vi "Read Protocol ID.vi"(8 "error in (no error)":errorcluster, 11 "MB_ADU_TCP in":refnum<class "MB_ADU_TCP.lvclass">) -> (0 "error out":errorcluster, 2 "Protocol ID":u16, 3 "MB_ADU_TCP out":refnum<class "MB_ADU_TCP.lvclass">)   [LabVIEW 2012, in "MB Master.lvlib" / "MB_ADU_TCP.lvclass"]
uses:
  MB_ADU_TCP.lvclass
  MB_ADU_TCP.lvclass/MB_ADU_TCP.ctl
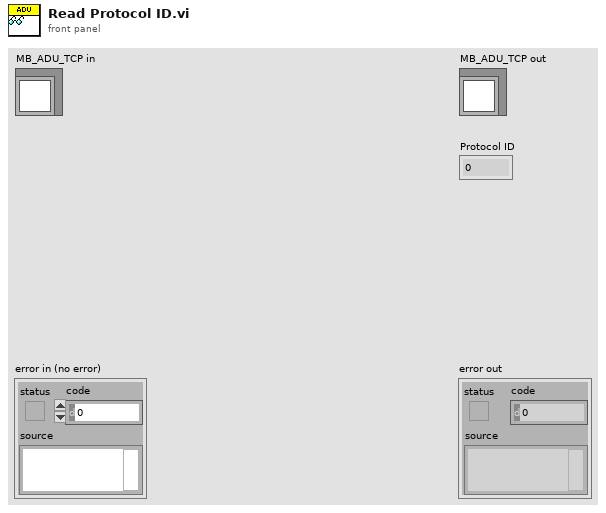
[diagram p1: front panel]
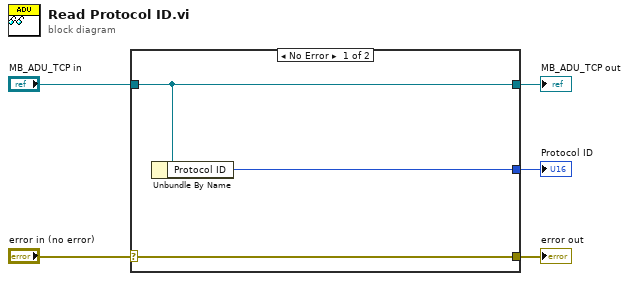
[diagram p0: block diagram]
diagram:
  n1 = case shown="No Error" "error in (no error)" {
    selector: "error in (no error)" -> [w8 w9]
    tunnel: [w8 w9] -> w4
    tunnel: [w7 w10] -> w2
    tunnel: "MB_ADU_TCP in" -> [w7 w10]
    tunnel: [w6 _] -> w1
    frame No Error {
      n2 = Unbundle By Name(w7) -> ("Protocol ID"=w6:u16)
    }
    frame Error {
    }
  }
  "error out" <- w4
  "MB_ADU_TCP out" <- w2
  "Protocol ID" <- w1
